vi "DHE_SaveIDparams.vi"(6 "autoid":string, 7 "expidcounter":i32, 10 "expidbase":string) -> ()   [LabVIEW 2016]
uses:
  <vilib>/Utility/config.llb/Write Key (String).vi
  <vilib>/Utility/config.llb/Write Key (I32).vi
  <vilib>/Utility/config.llb/NI_LVConfig.lvlib
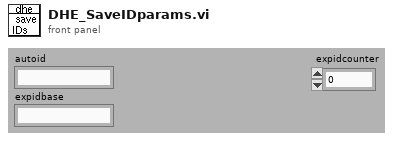
[diagram p1: front panel]
types:
  T1 = typedef "NI_LVConfig.lvlib/Config Data RefNum.ctl" = refnum<k1>
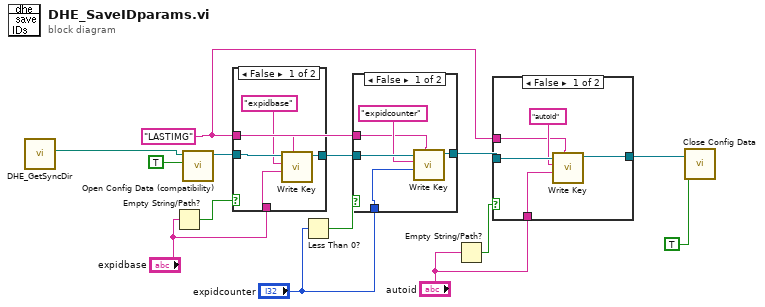
[diagram p0: block diagram]
diagram:
  w4 = "LASTIMG" ("section")
  n1 = call "DHE_GetSyncDir.vi"() -> ("sync file"=w1:path)  [unwired: 11 out]
  n2 = Empty String/Path?(string/path="expidbase") -> (empty?=w8:bool)
  n3 = call <vilib>:"Open Config Data (compatibility).vi"("create file if necessary (T)"=TRUE ("create file if necessary? (T)"), "configuration file path"=w1) -> ("refnum"=w14:T1)  [unwired: 7 in, 2 out]
  n4 = case shown="False" w8 {
    tunnel: w14 -> [w19 w20]
    tunnel: [w18 w20] -> w13
    tunnel: w4 -> [w16 _]
    tunnel: "expidbase" -> [w15 _]
    frame False {
      n5 = call-poly <vilib>:"Write Key.vi"("section"=w16, "value"=w15, "key"="expidbase", "refnum"=w19) -> ("refnum out"=w18:T1)  [unwired: 2 in, 5 out]
    }
    frame True {
    }
  }
  n6 = Less Than 0?(x="expidcounter") -> (x < 0?=w10:bool)
  n7 = case shown="False" w10 {
    tunnel: w13 -> [w25 w26]
    tunnel: [w24 w26] -> w6
    tunnel: w4 -> [w22 _]
    tunnel: "expidcounter" -> [w21 _]
    frame False {
      n8 = call-poly <vilib>:"Write Key.vi"("section"=w22, "value"=w21, "key"="expidcounter", "refnum"=w25) -> ("refnum out"=w24:T1)  [unwired: 1 in, 6 out]
    }
    frame True {
    }
  }
  n9 = Empty String/Path?(string/path="autoid") -> (empty?=w5:bool)
  n10 = case shown="False" w5 {
    tunnel: w6 -> [w31 w32]
    tunnel: [w30 w32] -> w3
    tunnel: w4 -> [w28 _]
    tunnel: "autoid" -> [w27 _]
    frame False {
      n11 = call-poly <vilib>:"Write Key.vi"("section"=w28, "value"=w27, "key"="autoid", "refnum"=w31) -> ("refnum out"=w30:T1)  [unwired: 2 in, 5 out]
    }
    frame True {
    }
  }
  n12 = call <vilib>:"Close Config Data.vi"("write file if changed (T)"=TRUE ("write configuration file? (T)"), "refnum"=w3) -> ()  [unwired: 1 in, 9 out]
